vi "c8855_calc_measurement_params_sub.vi"(3 "measurement params":T1, 4 "Gate time":i32, 5 "Measurement points":u32) -> (0 "measurement params out":T1)   [LabVIEW 2014]
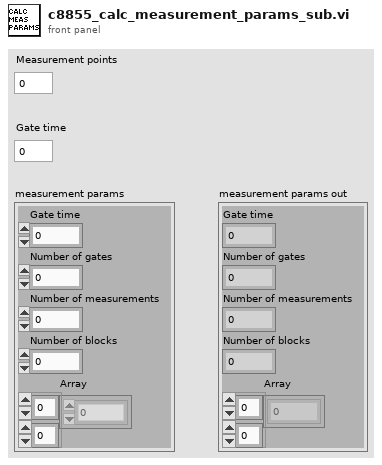
[diagram p1: front panel]
types:
  T1 = cluster{"Gate time":u8, "Number of gates":u16, "Number of measurements":i32, "Number of blocks":i32, "Array":u32[][]}
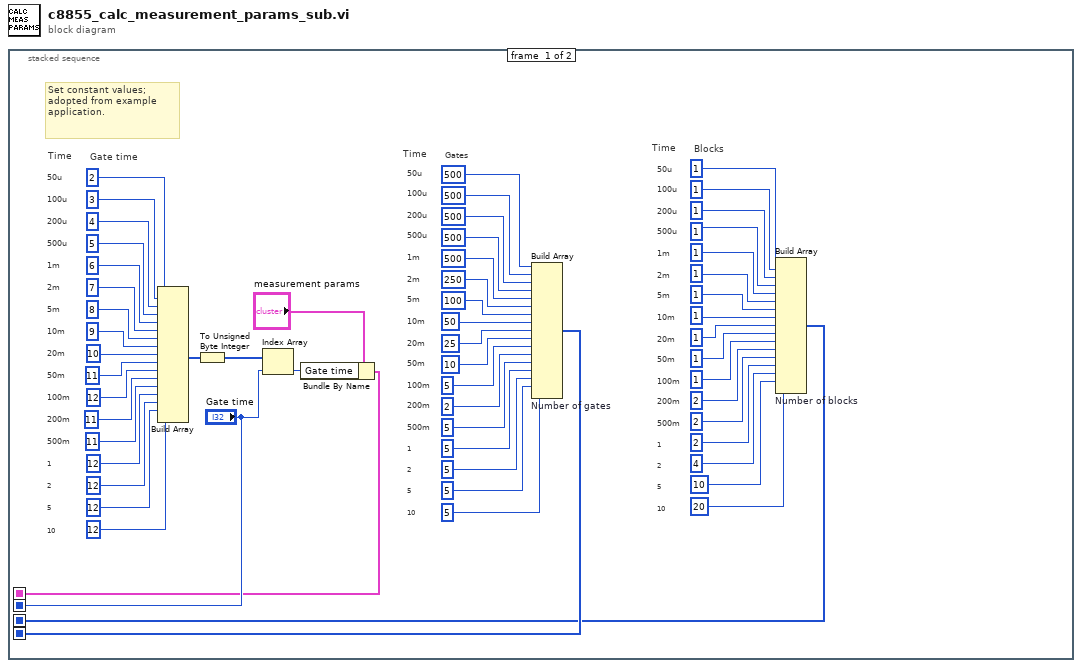
[diagram p0: block diagram]
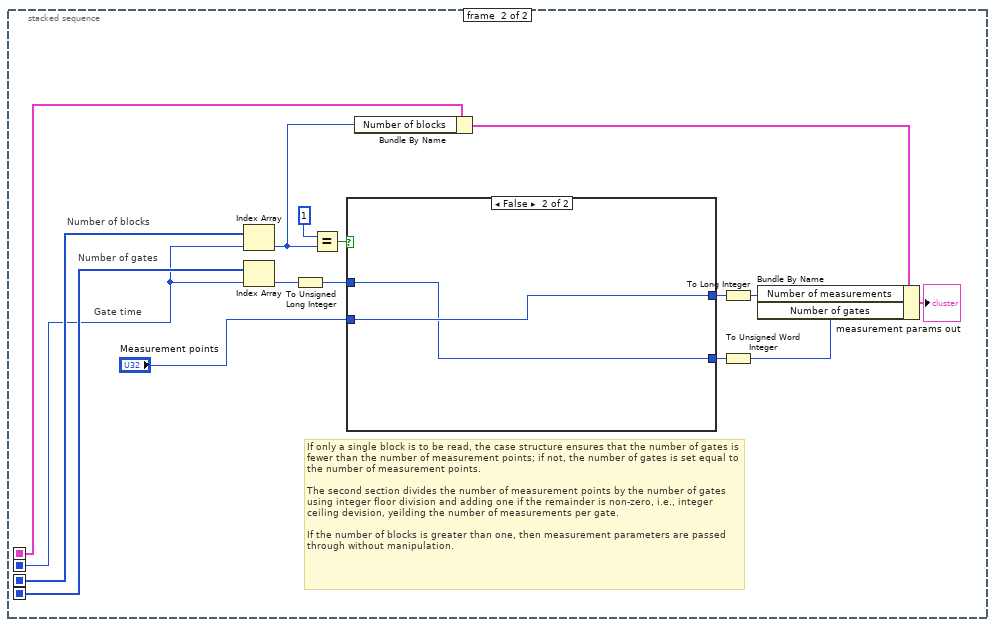
[diagram p2: hidden frame]
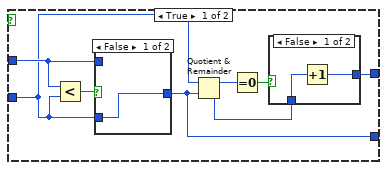
[diagram p3: hidden frame]
diagram:
  n1 = stacked-sequence {
    seq-local: [w1 _] -> [_ w65]
    seq-local: [w2 _] -> [_ w64]
    seq-local: [w3 _] -> [_ w63]
    seq-local: ["Gate time" _] -> [_ w62]
    frame #0 {
      # "Set constant values; adopted from example application."
      # "Gate time"
      # "Time"
      # "Blocks"
      # "Time"
      # "Gates"
      # "Time"
      # "10"
      # "5"
      # "2"
      # "1"
      # "500m"
      # "200m"
      # "100m"
      # "50m"
      # "20m"
      # "10m"
      # "5m"
      # "2m"
      # "1m"
      # "500u"
      # "200u"
      # "100u"
      # "50u"
      # "10"
      # "5"
      # "2"
      # "1"
      # "500m"
      # "200m"
      # "100m"
      # "50m"
      # "20m"
      # "10m"
      # "5m"
      # "2m"
      # "1m"
      # "500u"
      # "200u"
      # "100u"
      # "50u"
      # "10"
      # "5"
      # "2"
      # "1"
      # "500m"
      # "200m"
      # "100m"
      # "50m"
      # "20m"
      # "10m"
      # "5m"
      # "2m"
      # "1m"
      # "500u"
      # "200u"
      # "100u"
      # "50u"
      n2 = Build Array ("Gate time")(2, 3, 4, 5, 6, 7, 8, 9, 10, 11, 12, 11, 11, 12, 12, 12, 12) -> (w25:i32[])
      n3 = To Unsigned Byte Integer(number=w25) -> (unsigned 8bit integer=w7:u8[])
      n4 = Index Array(array=w7, index="Gate time") -> (element=w5:u8)
      n5 = Bundle By Name(cluster="measurement params", "Gate time"=w5) -> (w3:T1)
      n6 = Build Array "Number of gates"(u16 500, u16 500, u16 500, u16 500, u16 500, u16 250, u16 100, u16 50, u16 25, u16 10, u16 5, u16 2, u16 5, u16 5, u16 5, u16 5, u16 5) -> (w2:u16[])
      n7 = Build Array "Number of blocks"(1 ("SLoop"), 1 ("SLoop"), 1 ("SLoop"), 1 ("SLoop"), 1 ("SLoop"), 1 ("SLoop"), 1 ("SLoop"), 1 ("SLoop"), 1 ("SLoop"), 1 ("SLoop"), 1 ("SLoop"), 2 ("SLoop"), 2 ("SLoop"), 2 ("SLoop"), 4 ("SLoop"), 10 ("SLoop"), 20 ("SLoop")) -> (w1:i32[])
    }
    frame #1 {
      # "If only a single block is to be read, the case structure ensures that the number of gates is fewer than the number of measurement points; if not, the number of gates is set equal to the number of measurement points.\n\nThe second section divides the number of measurement points by the number of gates using integer floor division and adding one if the remainder is non-zero, i.e., integer ceiling devision, yeilding the number of measurements per gate.\n\nIf the number of blocks is greater than one, then measurement parameters are passed through without manipulation."
      # "Gate time"
      # "Number of blocks"
      # "Number of gates"
      n8 = Index Array(array=w65, index=w62) -> (element=w61:i32)
      n9 = Index Array(array=w64, index=w62) -> (element=w68:u16)
      n10 = To Unsigned Long Integer(number=w68) -> (unsigned 32bit integer=w67:u32)
      n11 = Equal?(x=1, y=w61) -> (x = y?=w74:bool)
      n12 = case shown="False" w74 {
        tunnel: [w77 w90] -> w73
        tunnel: w67 -> [w82 w89]
        tunnel: "Measurement points" -> [w81 w90]
        tunnel: [w76 w89] -> w70
        frame True {
          n13 = Less?(x=w82, y=w81) -> (x < y?=w83:bool)
          n14 = case shown="False" w83 {
            tunnel: w81 -> [w87 _]
            tunnel: w82 -> [_ w88]
            tunnel: [w87 w88] -> w76
            frame False {
            }
            frame True {
            }
          }
          n15 = Quotient & Remainder(x=w81, y=w76) -> (x-y*floor(x/y)=w80:u32, floor(x/y)=w78:u32)
          n16 = Equal To 0?(x=w80) -> (x = 0?=w79:bool)
          n17 = case shown="False" w79 {
            tunnel: w78 -> [w85 w86]
            tunnel: [w84 w86] -> w77
            frame False {
              n18 = Increment(x=w85) -> (x+1=w84:u32)
            }
            frame True {
            }
          }
        }
        frame False {
        }
      }
      n19 = Bundle By Name(cluster=w63, "Number of blocks"=w61) -> (w72:T1)
      n20 = To Long Integer(number=w73) -> (32bit integer=w71:i32)
      n21 = To Unsigned Word Integer(number=w70) -> (unsigned 16bit integer=w69:u16)
      n22 = Bundle By Name(cluster=w72, "Number of measurements"=w71, "Number of gates"=w69) -> (→"measurement params out":T1)
    }
  }
